vi "_setControlRef.vi"(7 "parentURL":string, 8 "error in (no error)":errorcluster, 9 "Name":string, 10 "Refnum":refnum<vi>, 11 "TagDB in":T1) -> (0 "error out":errorcluster, 2 "Ref-Key":string, 3 "TagDB out":T1)   [LabVIEW 2017, in "TagDB RefManager.lvlib"]
uses:
  TagDB RefManager.lvlib
  <userlib>/_NEVSTOP/TagDB/Typedef/TagDB.ctl
  39047c58-e22d-481c-91b5-4ba0bd035ec8.vi
  11f946b7-9f57-44fd-b0b0-69ef5a4d0f07.vi
  046b1344-6081-4f7d-b089-6eea8a81863f.vi
  <userlib>/_NEVSTOP/TagDB/_Support/DataAccess/data-Write.vi
  <userlib>/_NEVSTOP/TagDB/_Support/DataAccess/_NameCacher.vi
  <userlib>/_NEVSTOP/TagDB/_Support/DataAccess/_datatypeChecker.vi
  BlackList/_blacklist.vi
  <userlib>/_NEVSTOP/TagDB/_Support/DataAccess/TagDB Ref to DVR.vi
  <vilib>/Utility/Data Type/Get Type Information.vi
  <vilib>/Utility/error.llb/Trim Whitespace.vi
  <userlib>/_NEVSTOP/TagDB/_Support/Error/_[error50000]Invalid DB REF.vi
  <userlib>/_NEVSTOP/TagDB/TagDB.lvlib
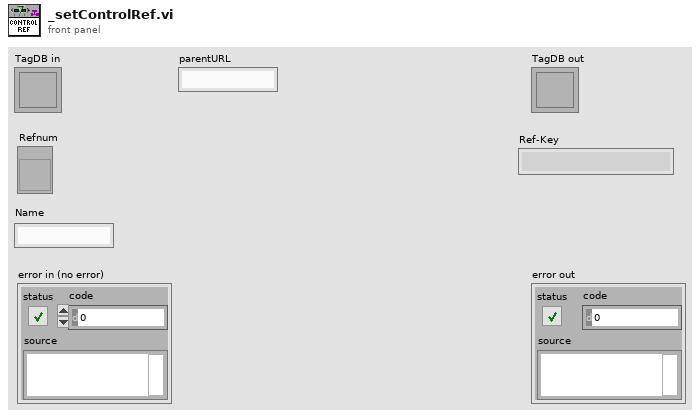
[diagram p1: front panel]
types:
  T1 = typedef "TagDB.lvlib/TagDB.ctl" = refnum<k1>
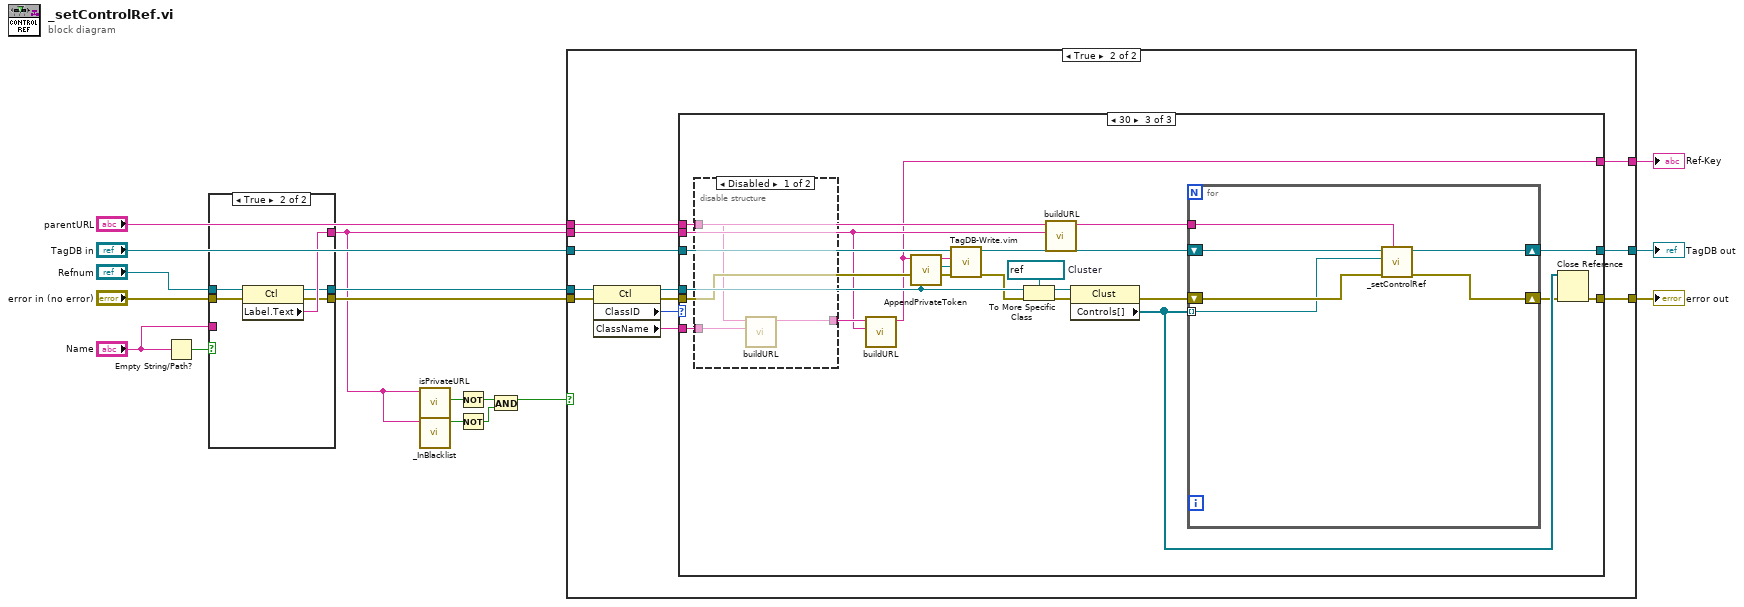
[diagram p0: block diagram]
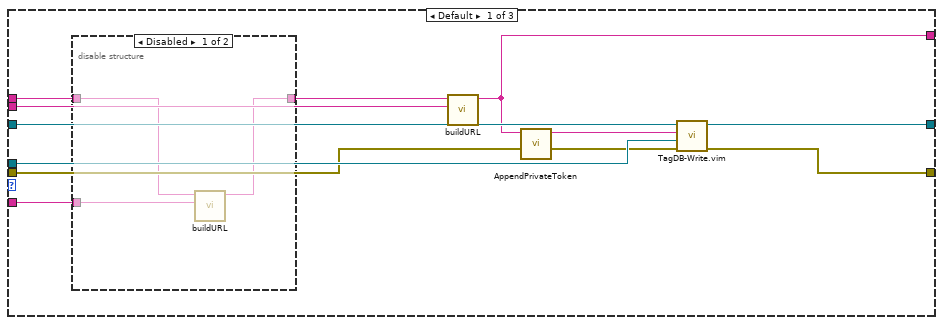
[diagram p3: hidden frame]
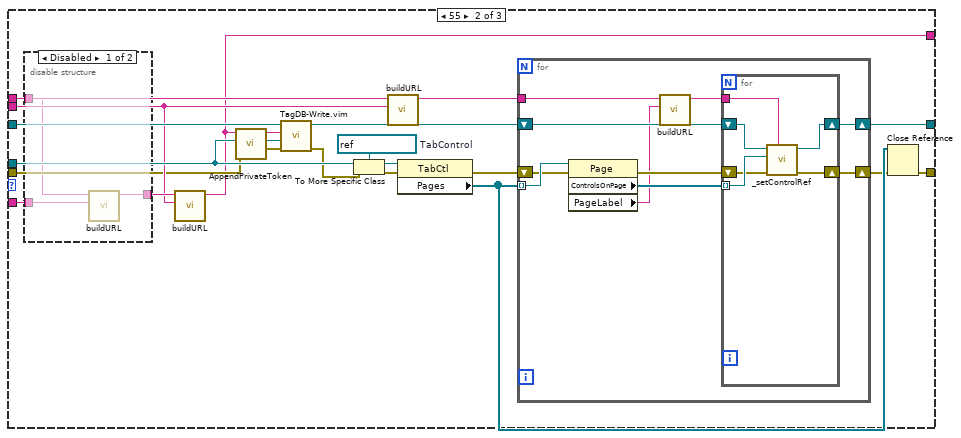
[diagram p5: hidden frame]
diagram:
  n1 = Empty String/Path?(string/path="Name") -> (empty?=w13:bool)
  n2 = case shown="True" w13 {
    tunnel: "error in (no error)" -> [w18 w25]
    tunnel: "Refnum" -> [w19 w24]
    tunnel: [w20 w23] -> w6
    tunnel: [w19 w22] -> w11
    tunnel: [w18 w21] -> w9
    tunnel: "Name" -> [w20 _]
    frame False {
    }
    frame True {
      n3 = property class="Ctl"(reference=w24, error in=w25) -> (reference out=w22:refnum<vi>, error out=w21:errorcluster, "Label.Text"=w23:string)
    }
  }
  n4 = call <userlib>:"isPrivateURL.vi"("URL"=w6) -> ("private?"=w1:bool)  [unwired: 9 in, 1 out]
  n5 = call "_InBlacklist.vi"("String"=w6) -> ("in blacklist?"=w3:bool)  [unwired: 10 in]
  n6 = Not(x=w1) -> (.not. x?=w4:bool)
  n7 = Not(x=w3) -> (.not. x?=w2:bool)
  n8 = And(x=w4, y=w2) -> (x .and. y?=w5:bool)
  n9 = case shown="True" w5 {
    tunnel: "parentURL" -> [w26 w40]
    tunnel: [w27 w36] -> w16
    tunnel: [w28 w35] -> w15
    tunnel: "TagDB in" -> [w28 w34]
    tunnel: w11 -> [_ w33]
    tunnel: w9 -> [w27 w32]
    tunnel: [w26 w31] -> w7
    tunnel: w6 -> [_ w30]
    frame False {
    }
    frame True {
      n10 = property on="Property Node" class="Ctl"(reference=w33, error in=w32) -> (reference out=w37:refnum<vi>, error out=w38:errorcluster, "ClassID"=w39:u32, "ClassName"=w29:string)
      n11 = case shown="30" w39 {
        tunnel: w34 -> [w49 w64 w106]
        tunnel: [w48 w69 w109] -> w35
        tunnel: w38 -> [w43 w59 w104]
        tunnel: [w42 w72 w112] -> w36
        tunnel: w37 -> [w44 w62 w105]
        tunnel: w40 -> [w50 w57 w101]
        tunnel: w30 -> [w47 w60 w99]
        tunnel: [w41 w56 w96] -> w31
        tunnel: w29 -> [w46 w61 w100]
        frame Default {
          n12 = disable-structure shown="Disabled" {
            disable-tunnel: [w54 w55] -> w51
            disable-tunnel: w50 -> [w53 w55]
            disable-tunnel: w46 -> [w52 _]
            frame Disabled {
              n13 = call <userlib>:"buildURL.vi"("DataName"=w52, "parentURL"=w53) -> ("DataURL"=w54:string)  [unwired: 9 in]
            }
            frame Enabled {
            }
          }
          n14 = call <userlib>:"buildURL.vi"("DataName"=w47, "parentURL"=w51) -> ("DataURL"=w41:string)  [unwired: 9 in]
          n15 = call <userlib>:"AppendPrivateToken.vi"("DataURL"=w41) -> ("String"=w45:string)  [unwired: 10 in]
          n16 = call "TagDB-Write.vim"("error in (no error)"=w43, "Value"=w44, "name"=w45, "TagDB"=w49) -> ("error out"=w42:errorcluster, "TagDB(dup)"=w48:T1)  [unwired: 5 in, 1 out]
        }
        frame 55 {
          w75 = refnum<vi> refnum  # TabControl
          n17 = disable-structure shown="Disabled" {
            disable-tunnel: [w78 w79] -> w66
            disable-tunnel: w61 -> [w77 _]
            disable-tunnel: w57 -> [w76 w79]
            frame Disabled {
              n18 = call <userlib>:"buildURL.vi"("DataName"=w77, "parentURL"=w76) -> ("DataURL"=w78:string)  [unwired: 9 in]
            }
            frame Enabled {
            }
          }
          n19 = call <userlib>:"buildURL.vi"("DataName"=w60, "parentURL"=w66) -> ("DataURL"=w56:string)  [unwired: 9 in]
          n20 = call <userlib>:"AppendPrivateToken.vi"("DataURL"=w56) -> ("String"=w65:string)  [unwired: 10 in]
          n21 = call "TagDB-Write.vim"("error in (no error)"=w59, "Value"=w62, "name"=w65, "TagDB"=w64) -> ("error out"=w58:errorcluster, "TagDB(dup)"=w63:T1)  [unwired: 5 in, 1 out]
          n22 = To More Specific Class(target class=w75, reference=w62, error in=w58) -> (specific class reference=w74:refnum<vi>, error out=w73:errorcluster)
          n23 = call <userlib>:"buildURL.vi"("DataName"=w60, "parentURL"=w57) -> ("DataURL"=w67:string)  [unwired: 9 in]
          n24 = property class="TabCtl"(reference=w74, error in=w73) -> (error out=w70:errorcluster, "Pages"=w71:refnum<vi>[])  [unwired: 1 out]
          n25 = for {
            tunnel: w71 -> [w89] mode=indexing
            shift-right: [w83] -> w68
            shift-left: w70 -> [w88]
            shift-right: [w85] -> w69
            shift-left: w63 -> [w86]
            tunnel: w67 -> [w81]
            n26 = property class="Page"(reference=w89, error in=w88) -> (error out=w84:errorcluster, "ControlsOnPage"=w87:refnum<vi>[], "PageLabel"=w80:string)  [unwired: 1 out]
            n27 = call <userlib>:"buildURL.vi"("DataName"=w80, "parentURL"=w81) -> ("DataURL"=w82:string)  [unwired: 9 in]
            n28 = for {
              tunnel: w87 -> [w95] mode=indexing
              shift-right: [w93] -> w85
              shift-left: w86 -> [w94]
              shift-right: [w91] -> w83
              shift-left: w84 -> [w92]
              tunnel: w82 -> [w90]
              n29 = call "_setControlRef.vi"("parentURL"=w90, "error in (no error)"=w92, "Refnum"=w95, "TagDB in"=w94) -> ("error out"=w91:errorcluster, "TagDB out"=w93:T1)  [unwired: 5 in, 1 out]
            }
          }
          n30 = Close Reference(reference=w71, error in (no error)=w68) -> (error out=w72:errorcluster)
        }
        frame 30 {
          w115 = refnum<vi> refnum  # Cluster
          n31 = disable-structure shown="Disabled" {
            disable-tunnel: [w118 w119] -> w102
            disable-tunnel: w101 -> [w117 w119]
            disable-tunnel: w100 -> [w116 _]
            frame Disabled {
              n32 = call <userlib>:"buildURL.vi"("DataName"=w116, "parentURL"=w117) -> ("DataURL"=w118:string)  [unwired: 9 in]
            }
            frame Enabled {
            }
          }
          n33 = call <userlib>:"buildURL.vi"("DataName"=w99, "parentURL"=w102) -> ("DataURL"=w96:string)  [unwired: 9 in]
          n34 = call <userlib>:"AppendPrivateToken.vi"("DataURL"=w96) -> ("String"=w98:string)  [unwired: 10 in]
          n35 = call "TagDB-Write.vim"("error in (no error)"=w104, "Value"=w105, "name"=w98, "TagDB"=w106) -> ("error out"=w103:errorcluster, "TagDB(dup)"=w97:T1)  [unwired: 5 in, 1 out]
          n36 = To More Specific Class(target class=w115, reference=w105, error in=w103) -> (specific class reference=w114:refnum<vi>, error out=w113:errorcluster)
          n37 = call <userlib>:"buildURL.vi"("DataName"=w99, "parentURL"=w101) -> ("DataURL"=w107:string)  [unwired: 9 in]
          n38 = property class="Clust"(reference=w114, error in=w113) -> (error out=w110:errorcluster, "Controls[]"=w111:refnum<vi>[])  [unwired: 1 out]
          n39 = for {
            tunnel: w111 -> [w120] mode=indexing
            shift-right: [w123] -> w108
            shift-left: w110 -> [w121]
            shift-right: [w124] -> w109
            shift-left: w97 -> [w125]
            tunnel: w107 -> [w122]
            n40 = call "_setControlRef.vi"("parentURL"=w122, "error in (no error)"=w121, "Refnum"=w120, "TagDB in"=w125) -> ("error out"=w123:errorcluster, "TagDB out"=w124:T1)  [unwired: 5 in, 1 out]
          }
          n41 = Close Reference(reference=w111, error in (no error)=w108) -> (error out=w112:errorcluster)
        }
      }
    }
  }
  "error out" <- w16
  "TagDB out" <- w15
  "Ref-Key" <- w7
